vi "PW_LDA analysis top level_PN.vi"() -> ()   [LabVIEW 2010]
uses:
  PW_LDA control cluster.ctl
  PW_LDA wrapper control cluster.ctl
  <vilib>/Utility/file.llb/Read From Spreadsheet File (string).vi
panel:
  out "Correl files creation error":errorcluster
  out "Correl files writing / closing error":errorcluster
  out "stats file error":errorcluster
  out "Final error":errorcluster
  out "No. of rows":i32=67
  in  "Stats output directory":path=path "C:/LDAPW data/5ms_stats"
  out "Current row no.":i32=2
  in  "Wrapper controls":T1={"N blocks"=20, "PW lag time start (s)"=-0.2, "PW lag time finish (s)"=0.2, "PW lag time dt (s)"=0.2, "Desired lag time for stats (s)"=0.0, "stats order"=4, "PDF(T) or hist(F)"=TRUE, "Nbins U"=32, "Nbins V"=32, "Mean shift"=FALSE, "2nd comp."="v"}
  out "Batch file":string[][](array[string])=[["Block data path", "Output directory for lagged correls.", "X (mm)", "Y (mm)", "N blocks"], ["NEXT", "C:\\LDAPW data\\x=0_5ms", "", "", ""], ["C:\\LDAPW data\\x=0, y=0.5 5ms", "C:\\LDAPW data\\x=0_5ms", "0", "0.5", "20"], ["C:\\LDAPW data\\x=0, y=0.79 5ms", "C:\\LDAPW data\\x=0_5ms", "0", "0.79", "20"], ["C:\\LDAPW data\\x=0, y=1.23 5ms", "C:\\LDAPW data\\x=0_5ms", "0", "1.23", "20"], ["C:\\LDAPW data\\x=0, y=1.94 5ms", "C:\\LDAPW data\\x=0_5ms", "0", "1.94", "20"], ["C:\\LDAPW data\\x=0, y=3.04 5ms", "C:\\LDAPW data\\x=0_5ms", "0", "3.04", "20"], ["C:\\LDAPW data\\x=0, y=4.78 5ms", "C:\\LDAPW data\\x=0_5ms", "0", "4.78", "20"], ["C:\\LDAPW data\\x=0, y=7.5 5ms", "C:\\LDAPW data\\x=0_5ms", "0", "7.5", "20"], ["NEXT", "C:\\LDAPW data\\x=20_5ms", "", "", ""], ["C:\\LDAPW data\\x=20, y=0.5 5ms", "C:\\LDAPW data\\x=20_5ms", "20", "0.5", "20"], ["C:\\LDAPW data\\x=20, y=0.79 5ms", "C:\\LDAPW data\\x=20_5ms", "20", "0.79", "20"], ["C:\\LDAPW data\\x=20, y=1.23 5ms", "C:\\LDAPW data\\x=20_5ms", "20", "1.23", "20"], ["C:\\LDAPW data\\x=20, y=1.94 5ms", "C:\\LDAPW data\\x=20_5ms", "20", "1.94", "20"], ["C:\\LDAPW data\\x=20, y=3.04 5ms", "C:\\LDAPW data\\x=20_5ms", "20", "3.04", "20"], ["C:\\LDAPW data\\x=20, y=4.78 5ms", "C:\\LDAPW data\\x=20_5ms", "20", "4.78", "20"], ["C:\\LDAPW data\\x=20, y=7.5 5ms", "C:\\LDAPW data\\x=20_5ms", "20", "7.5", "20"], ["NEXT", "C:\\LDAPW data\\x=40_5ms", "", "", ""], ["C:\\LDAPW data\\x=40, y=0.55 5ms", "C:\\LDAPW data\\x=40_5ms", "40", "0.55", "20"], ["C:\\LDAPW data\\x=40, y=0.79 5ms", "C:\\LDAPW data\\x=40_5ms", "40", "0.79", "20"], ["C:\\LDAPW data\\x=40, y=1.23 5ms", "C:\\LDAPW data\\x=40_5ms", "40", "1.23", "20"], ["C:\\LDAPW data\\x=40, y=1.94 5ms", "C:\\LDAPW data\\x=40_5ms", "40", "1.94", "20"], ["C:\\LDAPW data\\x=40, y=3.04 5ms", "C:\\LDAPW data\\x=40_5ms", "40", "3.04", "20"], ["C:\\LDAPW data\\x=40, y=4.78 5ms", "C:\\LDAPW data\\x=40_5ms", "40", "4.78", "20"], ["C:\\LDAPW data\\x=40, y=7.5 5ms", "C:\\LDAPW data\\x=40_5ms", "40", "7.5", "20"], ["NEXT", "C:\\LDAPW data\\x=60_5ms", "", "", ""], ["C:\\LDAPW data\\x=60, y=0.5 5ms", "C:\\LDAPW data\\x=60_5ms", "60", "0.5", "20"], ["C:\\LDAPW data\\x=60, y=0.79 5ms", "C:\\LDAPW data\\x=60_5ms", "60", "0.79", "20"], ["C:\\LDAPW data\\x=60, y=1.23 5ms", "C:\\LDAPW data\\x=60_5ms", "60", "1.23", "20"], ["C:\\LDAPW data\\x=60, y=1.94 5ms", "C:\\LDAPW data\\x=60_5ms", "60", "1.94", "20"], ["C:\\LDAPW data\\x=60, y=3.04 5ms", "C:\\LDAPW data\\x=60_5ms", "60", "3.04", "20"], ["C:\\LDAPW data\\x=60, y=4.78 5ms", "C:\\LDAPW data\\x=60_5ms", "60", "4.78", "20"], ["C:\\LDAPW data\\x=60, y=7.5 5ms", "C:\\LDAPW data\\x=60_5ms", "60", "7.5", "20"], ["NEXT", "C:\\LDAPW data\\x=80_5ms", "", "", ""], ["C:\\LDAPW data\\x=80, y=0.5 5ms", "C:\\LDAPW data\\x=80_5ms", "80", "0.5", "20"], ["C:\\LDAPW data\\x=80, y=0.79 5ms", "C:\\LDAPW data\\x=80_5ms", "80", "0.79", "20"], ["C:\\LDAPW data\\x=80, y=1.23 5ms", "C:\\LDAPW data\\x=80_5ms", "80", "1.23", "20"], ["C:\\LDAPW data\\x=80, y=1.94 5ms", "C:\\LDAPW data\\x=80_5ms", "80", "1.94", "20"], ["C:\\LDAPW data\\x=80, y=3.04 5ms", "C:\\LDAPW data\\x=80_5ms", "80", "3.04", "20"], ["C:\\LDAPW data\\x=80, y=4.78 5ms", "C:\\LDAPW data\\x=80_5ms", "80", "4.78", "20"], ["C:\\LDAPW data\\x=80, y=7.5 5ms", "C:\\LDAPW data\\x=80_5ms", "80", "7.5", "20"], ["NEXT", "C:\\LDAPW data\\x=100_5ms", "", "", ""], ["C:\\LDAPW data\\x=100, y=0.5 5ms", "C:\\LDAPW data\\x=100_5ms", "100", "0.5", "20"], ["C:\\LDAPW data\\x=100, y=0.79 5ms", "C:\\LDAPW data\\x=100_5ms", "100", "0.79", "20"], ["C:\\LDAPW data\\x=100, y=1.23 5ms", "C:\\LDAPW data\\x=100_5ms", "100", "1.23", "20"], ["C:\\LDAPW data\\x=100, y=1.94 5ms", "C:\\LDAPW data\\x=100_5ms", "100", "1.94", "20"], ["C:\\LDAPW data\\x=100, y=3.04 5ms", "C:\\LDAPW data\\x=100_5ms", "100", "3.04", "20"], ["C:\\LDAPW data\\x=100, y=4.78 5ms", "C:\\LDAPW data\\x=100_5ms", "100", "4.78", "20"], ["C:\\LDAPW data\\x=100, y=7.5 5ms", "C:\\LDAPW data\\x=100_5ms", "100", "7.5", "20"], ["NEXT", "C:\\LDAPW data\\x=120_5ms", "", "", ""], ["C:\\LDAPW data\\x=120, y=0.5 5ms", "C:\\LDAPW data\\x=120_5ms", "120", "0.5", "20"], ["C:\\LDAPW data\\x=120, y=0.79 5ms", "C:\\LDAPW data\\x=120_5ms", "120", "0.79", "20"], ["C:\\LDAPW data\\x=120, y=1.23 5ms", "C:\\LDAPW data\\x=120_5ms", "120", "1.23", "20"], ["C:\\LDAPW data\\x=120, y=1.94 5ms", "C:\\LDAPW data\\x=120_5ms", "120", "1.94", "20"], ["C:\\LDAPW data\\x=120, y=3.04 5ms", "C:\\LDAPW data\\x=120_5ms", "120", "3.04", "20"], ["C:\\LDAPW data\\x=120, y=4.78 5ms", "C:\\LDAPW data\\x=120_5ms", "120", "4.78", "20"], ["C:\\LDAPW data\\x=120, y=7.5 5ms", "C:\\LDAPW data\\x=120_5ms", "120", "7.5", "20"], ["NEXT", "C:\\LDAPW data\\x=140_5ms", "", "", ""], ["C:\\LDAPW data\\x=140, y=0.5 5ms", "C:\\LDAPW data\\x=140_5ms", "140", "0.5", "20"], ["C:\\LDAPW data\\x=140, y=0.79 5ms", "C:\\LDAPW data\\x=140_5ms", "140", "0.79", "20"], ["C:\\LDAPW data\\x=140, y=1.23 5ms", "C:\\LDAPW data\\x=140_5ms", "140", "1.23", "20"], ["C:\\LDAPW data\\x=140, y=1.94 5ms", "C:\\LDAPW data\\x=140_5ms", "140", "1.94", "20"], ["C:\\LDAPW data\\x=140, y=3.04 5ms", "C:\\LDAPW data\\x=140_5ms", "140", "3.04", "20"], ["C:\\LDAPW data\\x=140, y=4.78 5ms", "C:\\LDAPW data\\x=140_5ms", "140", "4.78", "20"], ["C:\\LDAPW data\\x=140, y=7.5 5ms", "C:\\LDAPW data\\x=140_5ms", "140", "7.5", "20"], ["NEXT", "C:\\LDAPW data\\x=161.5_5ms", "", "", ""], ["C:\\LDAPW data\\x=161.5, y=0.53 5ms", "C:\\LDAPW data\\x=161.5_5ms", "161.5", "0.53", "20"], ["C:\\LDAPW data\\x=161.5, y=0.79 5ms", "C:\\LDAPW data\\x=161.5_5ms", "161.5", "0.79", "2"]]
  in  "Batch-file name":path=path "C:/LDAPW data/Full DataList.txt"
  in  "PW_LDA control cluster":T2={"Block data directory"=path "C:/LDAPW data/x=0, y=0.5 5ms", "An samp. rate (Hz)"=5000.0, "PW sampling rate (Hz)"=10.0, "PW samples per block"=300, "High threshold (V)"=2.5, "An. data prefix"="Analogue_", "LDA data prefix"="LDA_", "PW data prefix"="PW_", "LDA arr. t. prefix"="LDA_arr_t_", "filename suffix"=".txt", "interp. method"=1, "PW hardware delay (s)"=0.00085, "PW timing TOF fraction (0..1)"=0.5, "- LDA V"=TRUE, "PW TOF prefix"="PW_TOF_", "- LDA U"=FALSE, "- PW"=FALSE, "format"="%.16f"} {"interp. method" items=["nearest", "linear", "spline", "cubic Hermite", "Lagrange"]}
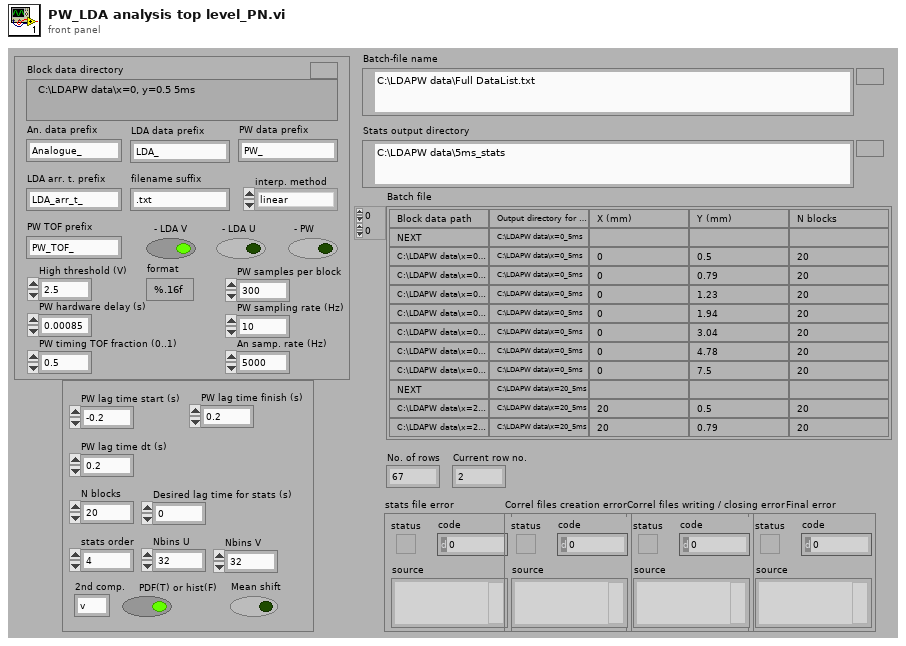
[diagram p1: front panel]
types:
  T1 = typedef "PW_LDA wrapper control cluster.ctl" = cluster{"N blocks":i32, "PW lag time start (s)":dbl, "PW lag time finish (s)":dbl, "PW lag time dt (s)":dbl, "Desired lag time for stats (s)":dbl, "stats order":i32, "PDF(T) or hist(F)":bool, "Nbins U":i32, "Nbins V":i32, "Mean shift":bool, "2nd comp.":string}
  T2 = typedef "PW_LDA control cluster.ctl" = cluster{"Block data directory":path, "An samp. rate (Hz)":dbl, "PW sampling rate (Hz)":dbl, "PW samples per block":i32, "High threshold (V)":dbl, "An. data prefix":string, "LDA data prefix":string, "PW data prefix":string, "LDA arr. t. prefix":string, "filename suffix":string, "interp. method":i32, "PW hardware delay (s)":dbl, "PW timing TOF fraction (0..1)":dbl, "- LDA V":bool, "PW TOF prefix":string, "- LDA U":bool, "- PW":bool, "format":string}
  T3 = enum16{"open", "replace", "create", "open or create", "replace or create", "replace or create with confirmation"}
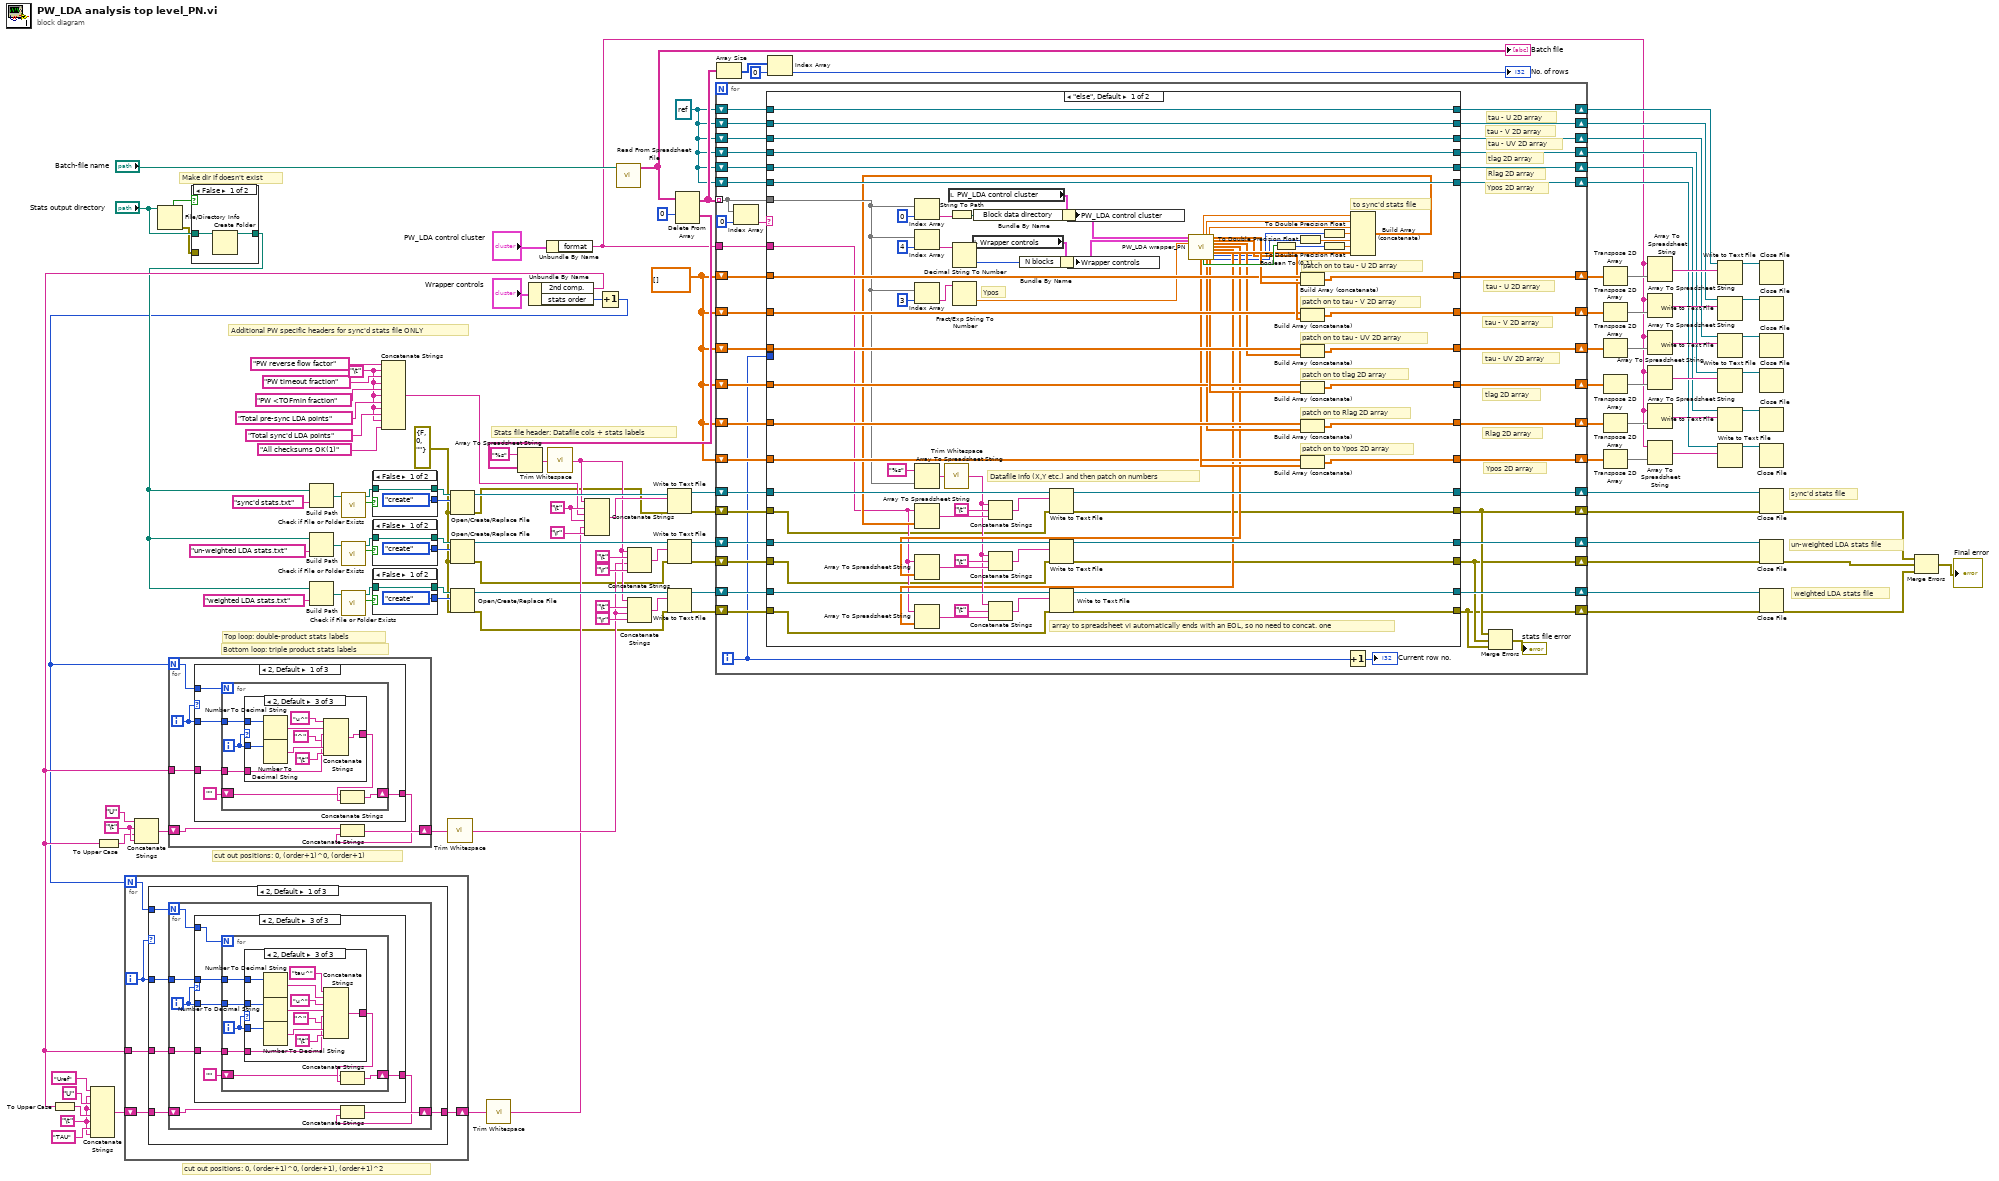
[diagram p0: block diagram]
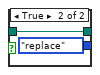
[diagram p3: hidden frame]
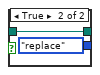
[diagram p4: hidden frame]
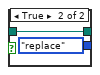
[diagram p5: hidden frame]
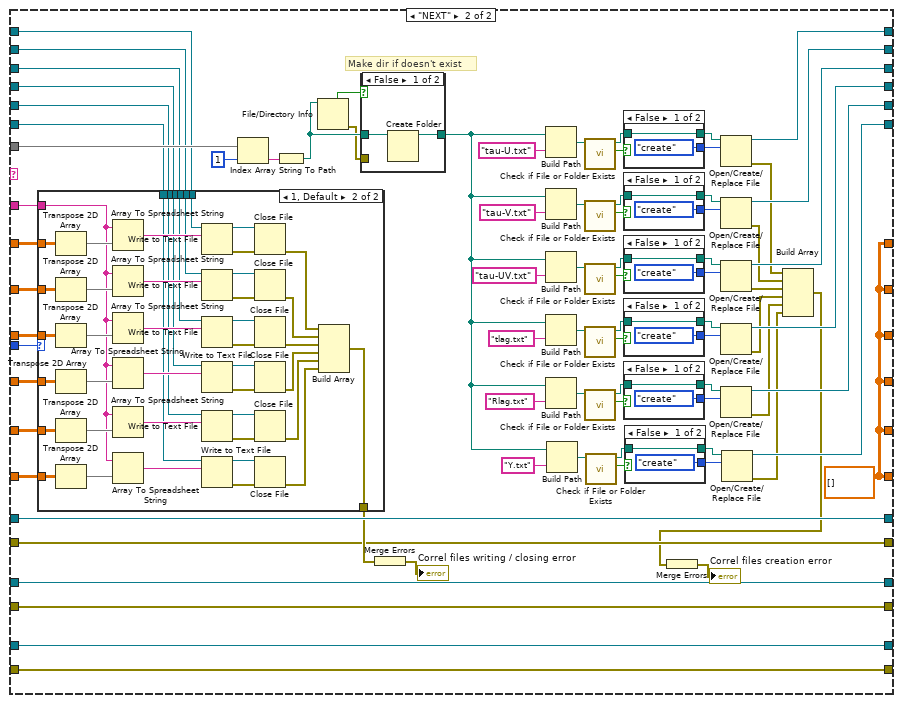
[diagram p6: hidden frame]
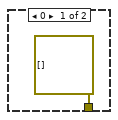
[diagram p8: hidden frame]
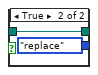
[diagram p9: hidden frame]
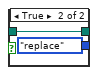
[diagram p10: hidden frame]
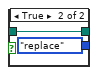
[diagram p11: hidden frame]
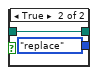
[diagram p12: hidden frame]
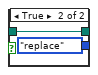
[diagram p13: hidden frame]
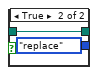
[diagram p14: hidden frame]
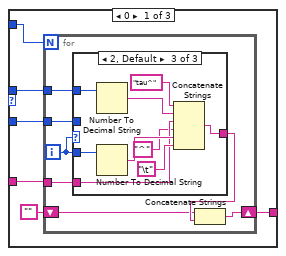
[diagram p15: hidden frame]
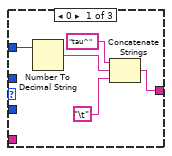
[diagram p16: hidden frame]
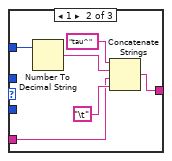
[diagram p17: hidden frame]
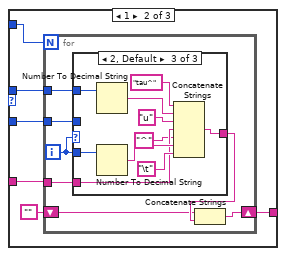
[diagram p18: hidden frame]
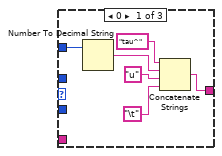
[diagram p19: hidden frame]
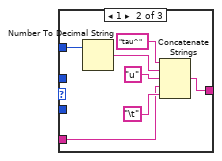
[diagram p20: hidden frame]
diagram:
  w14 = errorcluster {"status"=FALSE, "code"=0, "source"=""} ("error in")
  w64 = "\t"
  w70 = "\t"
  w112 = refnum<file> refnum ("refnum out")
  w111 = dbl[][] []
  w2 = "\t"
  w124 = "\t"
  # "Make dir if doesn't exist"
  # "Additional PW specific headers for sync'd stats file ONLY"
  # "Bottom loop: triple product stats labels"
  # "Top loop: double-product stats labels"
  # "Stats file header: Datafile cols + stats labels"
  # "weighted LDA stats file"
  # "un-weighted LDA stats file"
  # "sync'd stats file"
  # "cut out positions: 0, (order+1)^0, (order+1), (order+1)^2"
  # "cut out positions: 0, (order+1)^0, (order+1)"
  n1 = File/Directory Info(path="Stats output directory") -> (directory=w10:bool, error out=w7:errorcluster)  [unwired: 1 in, 5 out]
  n2 = case shown="False" w10 {
    tunnel: "Stats output directory" -> [w127 w128]
    tunnel: [w126 w128] -> w8
    tunnel: w7 -> [_ _]
    frame False {
      n3 = Create Folder(path (use dialog)=w127) -> (created path=w126:path)  [unwired: 1 in, 3 out]
    }
    frame True {
    }
  }
  n4 = Build Path(base path=w8, name or relative path="sync'd stats.txt" ("format string")) -> (appended path=w13:path)
  n5 = Build Path(base path=w8, name or relative path="un-weighted LDA stats.txt" ("format string")) -> (appended path=w12:path)
  n6 = Build Path(base path=w8, name or relative path="weighted LDA stats.txt" ("format string")) -> (appended path=w11:path)
  n7 = call <vilib>:"Check if File or Folder Exists.vi"("path"=w13) -> ("file or folder exists?"=w106:bool, "dup path"=w104:path)  [unwired: 1 in, 8 out]
  n8 = call <vilib>:"Check if File or Folder Exists.vi"("path"=w12) -> ("file or folder exists?"=w99:bool, "dup path"=w101:path)  [unwired: 1 in, 8 out]
  n9 = call <vilib>:"Check if File or Folder Exists.vi"("path"=w11) -> ("file or folder exists?"=w96:bool, "dup path"=w94:path)  [unwired: 1 in, 8 out]
  n10 = case shown="False" w106 {
    tunnel: [T3."create" ("operation (0:open)") T3."replace" ("operation (0:open)")] -> w105
    tunnel: [w129 w131] -> w103
    tunnel: w104 -> [w129 w131]
    frame False {
    }
    frame True {
    }
  }
  n11 = case shown="False" w99 {
    tunnel: [T3."create" ("operation (0:open)") T3."replace" ("operation (0:open)")] -> w100
    tunnel: [w133 w135] -> w102
    tunnel: w101 -> [w133 w135]
    frame False {
    }
    frame True {
    }
  }
  n12 = case shown="False" w96 {
    tunnel: [T3."create" ("operation (0:open)") T3."replace" ("operation (0:open)")] -> w95
    tunnel: [w137 w139] -> w93
    tunnel: w94 -> [w137 w139]
    frame False {
    }
    frame True {
    }
  }
  n13 = Concatenate Strings("PW reverse flow factor" ("format string"), w64, "PW timeout fraction" ("format string"), w64, "PW <TOFmin fraction" ("format string"), w64, "Total pre-sync LDA points" ("format string"), w64, "Total sync'd LDA points" ("format string"), w64, "All checksums OK(1)" ("format string")) -> (w62:string)
  n14 = Open/Create/Replace File(file path (use dialog)=w103, error in=w14, operation (0:open)=w105) -> (refnum out=w78:refnum<file>, error out=w59:errorcluster)  [unwired: 4 out]
  n15 = Open/Create/Replace File(file path (use dialog)=w102, error in=w14, operation (0:open)=w100) -> (refnum out=w77:refnum<file>, error out=w60:errorcluster)  [unwired: 4 out]
  n16 = Open/Create/Replace File(file path (use dialog)=w93, error in=w14, operation (0:open)=w95) -> (refnum out=w76:refnum<file>, error out=w61:errorcluster)  [unwired: 4 out]
  n17 = Unbundle By Name("Wrapper controls") -> ("2nd comp."=w108:string, "stats order"=w6:i32)
  n18 = To Upper Case(1:w108) -> (0:w4:string)
  n19 = Concatenate Strings("Uref" ("string"), w2, "U" ("string"), w2, w4, w2, "TAU" ("string"), w2) -> (w121:string)
  n20 = To Upper Case(1:w108) -> (0:w122:string)
  n21 = Concatenate Strings("U" ("string"), w124, w122, w124) -> (w123:string)
  n22 = Unbundle By Name("PW_LDA control cluster") -> ("format"=w22:string)
  n23 = Increment(x=w6) -> (x+1=w5:i32)
  n24 = for {
    N: w5 -> [w143]
    tunnel: w108 -> [w145]
    shift-right: [w144] -> w72
    shift-left: w121 -> [w142]
    i -> [w141]
    n25 = case shown="2, Default" w141 {
      tunnel: w145 -> [w150 w273 w363]
      tunnel: [w149 w272 w362] -> w144
      tunnel: w143 -> [w148 w271 w361]
      tunnel: w142 -> [w147 w270 w360]
      tunnel: w141 -> [w146 w269 w359]
      frame 2, Default {
        n26 = for {
          N: w148 -> [w157]
          shift-right: [w156] -> w149
          shift-left: w147 -> [w155]
          tunnel: w150 -> [w153]
          tunnel: w146 -> [w151]
          i -> [w152]
          n27 = case shown="2, Default" w152 {
            tunnel: w157 -> [w163 w196 w232]
            tunnel: [w161 w194 w230] -> w154
            tunnel: w153 -> [w160 w193 w229]
            tunnel: w152 -> [w159 w192 w228]
            tunnel: w151 -> [w158 w191 w227]
            frame 0 {
              n28 = for {
                N: w163 -> [_]
                shift-right: [w169] -> w161
                shift-left: "" -> [w168]
                tunnel: w159 -> [w167]
                tunnel: w160 -> [w166]
                tunnel: w158 -> [w164]
                i -> [w165]
                n29 = case shown="2, Default" w165 {
                  tunnel: [w175 w181 w190] -> w170
                  tunnel: w167 -> [_ _ _]
                  tunnel: w166 -> [_ w179 w187]
                  tunnel: w165 -> [_ _ w186]
                  tunnel: w164 -> [w173 w177 w184]
                  frame 0 {
                    n30 = Number To Decimal String(number=w173) -> (decimal integer string=w172:string)  [unwired: 1 out]
                    n31 = Concatenate Strings("tau^" ("t"), w172, "\t") -> (w175:string)
                  }
                  frame 1 {
                    n32 = Number To Decimal String(number=w177) -> (decimal integer string=w176:string)  [unwired: 1 out]
                    n33 = Concatenate Strings("tau^" ("t"), w176, w179, "\t") -> (w181:string)
                  }
                  frame 2, Default {
                    n34 = Number To Decimal String(number=w184) -> (decimal integer string=w183:string)  [unwired: 1 out]
                    n35 = Number To Decimal String(number=w186) -> (decimal integer string=w189:string)  [unwired: 1 out]
                    n36 = Concatenate Strings("tau^" ("t"), w183, w187, "^" ("string"), w189, "\t") -> (w190:string)
                  }
                }
                n37 = Concatenate Strings(w168, w170) -> (w169:string)
              }
            }
            frame 1 {
              n38 = for {
                N: w196 -> [_]
                shift-right: [w202] -> w194
                shift-left: "" -> [w201]
                tunnel: w192 -> [w200]
                tunnel: w193 -> [w199]
                tunnel: w191 -> [w197]
                i -> [w198]
                n39 = case shown="2, Default" w198 {
                  tunnel: [w208 w215 w225] -> w203
                  tunnel: w200 -> [_ _ _]
                  tunnel: w199 -> [_ w213 w222]
                  tunnel: w198 -> [_ _ w221]
                  tunnel: w197 -> [w206 w211 w219]
                  frame 0 {
                    n40 = Number To Decimal String(number=w206) -> (decimal integer string=w205:string)  [unwired: 1 out]
                    n41 = Concatenate Strings("tau^" ("t"), w205, "u" ("t"), "\t") -> (w208:string)
                  }
                  frame 1 {
                    n42 = Number To Decimal String(number=w211) -> (decimal integer string=w210:string)  [unwired: 1 out]
                    n43 = Concatenate Strings("tau^" ("t"), w210, "u" ("t"), w213, "\t") -> (w215:string)
                  }
                  frame 2, Default {
                    n44 = Number To Decimal String(number=w219) -> (decimal integer string=w218:string)  [unwired: 1 out]
                    n45 = Number To Decimal String(number=w221) -> (decimal integer string=w224:string)  [unwired: 1 out]
                    n46 = Concatenate Strings("tau^" ("t"), w218, "u" ("t"), w222, "^" ("string"), w224, "\t") -> (w225:string)
                  }
                }
                n47 = Concatenate Strings(w201, w203) -> (w202:string)
              }
            }
            frame 2, Default {
              n48 = for {
                N: w232 -> [_]
                shift-right: [w238] -> w230
                shift-left: "" -> [w237]
                tunnel: w228 -> [w236]
                tunnel: w229 -> [w235]
                tunnel: w227 -> [w233]
                i -> [w234]
                n49 = case shown="2, Default" w234 {
                  tunnel: [w246 w255 w267] -> w239
                  tunnel: w236 -> [w244 w253 w264]
                  tunnel: w235 -> [_ w251 w262]
                  tunnel: w234 -> [_ _ w261]
                  tunnel: w233 -> [w242 w249 w259]
                  frame 0 {
                    n50 = Number To Decimal String(number=w242) -> (decimal integer string=w241:string)  [unwired: 1 out]
                    n51 = Number To Decimal String(number=w244) -> (decimal integer string=w245:string)  [unwired: 1 out]
                    n52 = Concatenate Strings("tau^" ("t"), w241, "u^" ("t"), w245, "\t") -> (w246:string)
                  }
                  frame 1 {
                    n53 = Number To Decimal String(number=w249) -> (decimal integer string=w248:string)  [unwired: 1 out]
                    n54 = Number To Decimal String(number=w253) -> (decimal integer string=w254:string)  [unwired: 1 out]
                    n55 = Concatenate Strings("tau^" ("t"), w248, "u^" ("t"), w254, w251, "\t") -> (w255:string)
                  }
                  frame 2, Default {
                    n56 = Number To Decimal String(number=w259) -> (decimal integer string=w258:string)  [unwired: 1 out]
                    n57 = Number To Decimal String(number=w264) -> (decimal integer string=w266:string)  [unwired: 1 out]
                    n58 = Number To Decimal String(number=w261) -> (decimal integer string=w265:string)  [unwired: 1 out]
                    n59 = Concatenate Strings("tau^" ("t"), w258, "u^" ("t"), w266, w262, "^" ("string"), w265, "\t") -> (w267:string)
                  }
                }
                n60 = Concatenate Strings(w237, w239) -> (w238:string)
              }
            }
          }
          n61 = Concatenate Strings(w155, w154) -> (w156:string)
        }
      }
      frame 0 {
        n62 = for {
          N: w271 -> [w280]
          shift-right: [w279] -> w272
          shift-left: w270 -> [w278]
          tunnel: w273 -> [w276]
          tunnel: w269 -> [w274]
          i -> [w275]
          n63 = case shown="2, Default" w275 {
            tunnel: w280 -> [w286 w306 w331]
            tunnel: [w284 w304 w329] -> w277
            tunnel: w276 -> [w283 w303 w328]
            tunnel: w275 -> [w282 w302 w327]
            tunnel: w274 -> [w281 w301 w326]
            frame 0 {
              n64 = for {
                N: w286 -> [_]
                shift-right: [w292] -> w284
                shift-left: "" -> [w291]
                tunnel: w282 -> [w290]
                tunnel: w283 -> [w289]
                tunnel: w281 -> [w287]
                i -> [w288]
                n65 = case shown="2, Default" w288 {
                  tunnel: ["" w300] -> w293
                  tunnel: w290 -> [_ _]
                  tunnel: w289 -> [_ w297]
                  tunnel: w288 -> [_ w296]
                  tunnel: w287 -> [_ _]
                  frame 0, 1 {
                  }
                  frame 2, Default {
                    n66 = Number To Decimal String(number=w296) -> (decimal integer string=w299:string)  [unwired: 1 out]
                    n67 = Concatenate Strings(w297, "^" ("string"), w299, "\t") -> (w300:string)
                  }
                }
                n68 = Concatenate Strings(w291, w293) -> (w292:string)
              }
            }
            frame 1 {
              n69 = for {
                N: w306 -> [_]
                shift-right: [w312] -> w304
                shift-left: "" -> [w311]
                tunnel: w302 -> [w310]
                tunnel: w303 -> [w309]
                tunnel: w301 -> [w307]
                i -> [w308]
                n70 = case shown="2, Default" w308 {
                  tunnel: ["" w317 w324] -> w313
                  tunnel: w310 -> [_ _ _]
                  tunnel: w309 -> [_ w315 w321]
                  tunnel: w308 -> [_ _ w320]
                  tunnel: w307 -> [_ _ _]
                  frame 0 {
                  }
                  frame 1 {
                    n71 = Concatenate Strings("u" ("t"), w315, "\t") -> (w317:string)
                  }
                  frame 2, Default {
                    n72 = Number To Decimal String(number=w320) -> (decimal integer string=w323:string)  [unwired: 1 out]
                    n73 = Concatenate Strings("u" ("t"), w321, "^" ("string"), w323, "\t") -> (w324:string)
                  }
                }
                n74 = Concatenate Strings(w311, w313) -> (w312:string)
              }
            }
            frame 2, Default {
              n75 = for {
                N: w331 -> [_]
                shift-right: [w337] -> w329
                shift-left: "" -> [w336]
                tunnel: w327 -> [w335]
                tunnel: w328 -> [w334]
                tunnel: w326 -> [w332]
                i -> [w333]
                n76 = case shown="2, Default" w333 {
                  tunnel: [w342 w348 w357] -> w338
                  tunnel: w335 -> [w340 w346 w354]
                  tunnel: w334 -> [_ w344 w352]
                  tunnel: w333 -> [_ _ w351]
                  tunnel: w332 -> [_ _ _]
                  frame 0 {
                    n77 = Number To Decimal String(number=w340) -> (decimal integer string=w341:string)  [unwired: 1 out]
                    n78 = Concatenate Strings("u^" ("t"), w341, "\t") -> (w342:string)
                  }
                  frame 1 {
                    n79 = Number To Decimal String(number=w346) -> (decimal integer string=w347:string)  [unwired: 1 out]
                    n80 = Concatenate Strings("u^" ("t"), w347, w344, "\t") -> (w348:string)
                  }
                  frame 2, Default {
                    n81 = Number To Decimal String(number=w354) -> (decimal integer string=w356:string)  [unwired: 1 out]
                    n82 = Number To Decimal String(number=w351) -> (decimal integer string=w355:string)  [unwired: 1 out]
                    n83 = Concatenate Strings("u^" ("t"), w356, w352, "^" ("string"), w355, "\t") -> (w357:string)
                  }
                }
                n84 = Concatenate Strings(w336, w338) -> (w337:string)
              }
            }
          }
          n85 = Concatenate Strings(w278, w277) -> (w279:string)
        }
      }
      frame 1 {
        n86 = for {
          N: w361 -> [w370]
          shift-right: [w369] -> w362
          shift-left: w360 -> [w368]
          tunnel: w363 -> [w366]
          tunnel: w359 -> [w364]
          i -> [w365]
          n87 = case shown="2, Default" w365 {
            tunnel: w370 -> [w376 w401 w431]
            tunnel: [w375 w399 w429] -> w367
            tunnel: w366 -> [w374 w398 w428]
            tunnel: w365 -> [w373 w397 w427]
            tunnel: w364 -> [w372 w396 w426]
            frame 0 {
              n88 = for {
                N: w376 -> [_]
                shift-right: [w382] -> w375
                shift-left: "" -> [w381]
                tunnel: w373 -> [w380]
                tunnel: w374 -> [w379]
                tunnel: w372 -> [w377]
                i -> [w378]
                n89 = case shown="2, Default" w378 {
                  tunnel: ["" w388 w395] -> w383
                  tunnel: w380 -> [_ _ _]
                  tunnel: w379 -> [_ w386 w392]
                  tunnel: w378 -> [_ _ w391]
                  tunnel: w377 -> [_ _ _]
                  frame 0 {
                  }
                  frame 1 {
                    n90 = Concatenate Strings("tau" ("t"), w386, "\t") -> (w388:string)
                  }
                  frame 2, Default {
                    n91 = Number To Decimal String(number=w391) -> (decimal integer string=w394:string)  [unwired: 1 out]
                    n92 = Concatenate Strings("tau" ("t"), w392, "^" ("string"), w394, "\t") -> (w395:string)
                  }
                }
                n93 = Concatenate Strings(w381, w383) -> (w382:string)
              }
            }
            frame 1 {
              n94 = for {
                N: w401 -> [_]
                shift-right: [w407] -> w399
                shift-left: "" -> [w406]
                tunnel: w397 -> [w405]
                tunnel: w398 -> [w404]
                tunnel: w396 -> [w402]
                i -> [w403]
                n95 = case shown="2, Default" w403 {
                  tunnel: [w411 w416 w424] -> w408
                  tunnel: w405 -> [_ _ _]
                  tunnel: w404 -> [_ w414 w421]
                  tunnel: w403 -> [_ _ w420]
                  tunnel: w402 -> [_ _ _]
                  frame 0 {
                    n96 = Concatenate Strings("tau" ("t"), "u" ("t"), "\t") -> (w411:string)
                  }
                  frame 1 {
                    n97 = Concatenate Strings("tau" ("t"), "u" ("t"), w414, "\t") -> (w416:string)
                  }
                  frame 2, Default {
                    n98 = Number To Decimal String(number=w420) -> (decimal integer string=w423:string)  [unwired: 1 out]
                    n99 = Concatenate Strings("tau" ("t"), "u" ("t"), w421, "^" ("string"), w423, "\t") -> (w424:string)
                  }
                }
                n100 = Concatenate Strings(w406, w408) -> (w407:string)
              }
            }
            frame 2, Default {
              n101 = for {
                N: w431 -> [_]
                shift-right: [w437] -> w429
                shift-left: "" -> [w436]
                tunnel: w427 -> [w435]
                tunnel: w428 -> [w434]
                tunnel: w426 -> [w432]
                i -> [w433]
                n102 = case shown="2, Default" w433 {
                  tunnel: [w443 w450 w460] -> w438
                  tunnel: w435 -> [w441 w448 w457]
                  tunnel: w434 -> [_ w446 w455]
                  tunnel: w433 -> [_ _ w454]
                  tunnel: w432 -> [_ _ _]
                  frame 0 {
                    n103 = Number To Decimal String(number=w441) -> (decimal integer string=w442:string)  [unwired: 1 out]
                    n104 = Concatenate Strings("tau" ("t"), "u^" ("t"), w442, "\t") -> (w443:string)
                  }
                  frame 1 {
                    n105 = Number To Decimal String(number=w448) -> (decimal integer string=w449:string)  [unwired: 1 out]
                    n106 = Concatenate Strings("tau" ("t"), "u^" ("t"), w449, w446, "\t") -> (w450:string)
                  }
                  frame 2, Default {
                    n107 = Number To Decimal String(number=w457) -> (decimal integer string=w459:string)  [unwired: 1 out]
                    n108 = Number To Decimal String(number=w454) -> (decimal integer string=w458:string)  [unwired: 1 out]
                    n109 = Concatenate Strings("tau" ("t"), "u^" ("t"), w459, w455, "^" ("string"), w458, "\t") -> (w460:string)
                  }
                }
                n110 = Concatenate Strings(w436, w438) -> (w437:string)
              }
            }
          }
          n111 = Concatenate Strings(w368, w367) -> (w369:string)
        }
      }
    }
  }
  n112 = for {
    N: w5 -> [w467]
    shift-right: [w466] -> w74
    shift-left: w123 -> [w465]
    tunnel: w108 -> [w463]
    i -> [w462]
    n113 = case shown="2, Default" w462 {
      tunnel: w467 -> [w472 w503 w521]
      tunnel: [w470 w501 w519] -> w464
      tunnel: w463 -> [w469 w500 w518]
      tunnel: w462 -> [w468 w499 w517]
      frame 2, Default {
        n114 = for {
          N: w472 -> [_]
          shift-right: [w477] -> w470
          shift-left: "" -> [w476]
          tunnel: w468 -> [w475]
          tunnel: w469 -> [w474]
          i -> [w473]
          n115 = case shown="2, Default" w473 {
            tunnel: [w482 w488 w497] -> w478
            tunnel: w475 -> [w480 w486 w494]
            tunnel: w474 -> [_ w484 w492]
            tunnel: w473 -> [_ _ w491]
            frame 0 {
              n116 = Number To Decimal String(number=w480) -> (decimal integer string=w481:string)  [unwired: 1 out]
              n117 = Concatenate Strings("u^" ("t"), w481, "\t") -> (w482:string)
            }
            frame 1 {
              n118 = Number To Decimal String(number=w486) -> (decimal integer string=w487:string)  [unwired: 1 out]
              n119 = Concatenate Strings("u^" ("t"), w487, w484, "\t") -> (w488:string)
            }
            frame 2, Default {
              n120 = Number To Decimal String(number=w494) -> (decimal integer string=w496:string)  [unwired: 1 out]
              n121 = Number To Decimal String(number=w491) -> (decimal integer string=w495:string)  [unwired: 1 out]
              n122 = Concatenate Strings("u^" ("t"), w496, w492, "^" ("string"), w495, "\t") -> (w497:string)
            }
          }
          n123 = Concatenate Strings(w476, w478) -> (w477:string)
        }
      }
      frame 0 {
        n124 = for {
          N: w503 -> [_]
          shift-right: [w508] -> w501
          shift-left: "" -> [w507]
          tunnel: w499 -> [w506]
          tunnel: w500 -> [w505]
          i -> [w504]
          n125 = case shown="2, Default" w504 {
            tunnel: ["" w516] -> w509
            tunnel: w506 -> [_ _]
            tunnel: w505 -> [_ w513]
            tunnel: w504 -> [_ w512]
            frame 0, 1 {
            }
            frame 2, Default {
              n126 = Number To Decimal String(number=w512) -> (decimal integer string=w515:string)  [unwired: 1 out]
              n127 = Concatenate Strings(w513, "^" ("string"), w515, "\t") -> (w516:string)
            }
          }
          n128 = Concatenate Strings(w507, w509) -> (w508:string)
        }
      }
      frame 1 {
        n129 = for {
          N: w521 -> [_]
          shift-right: [w526] -> w519
          shift-left: "" -> [w525]
          tunnel: w517 -> [w524]
          tunnel: w518 -> [w523]
          i -> [w522]
          n130 = case shown="2, Default" w522 {
            tunnel: ["" w531 w538] -> w527
            tunnel: w524 -> [_ _ _]
            tunnel: w523 -> [_ w529 w535]
            tunnel: w522 -> [_ _ w534]
            frame 0 {
            }
            frame 1 {
              n131 = Concatenate Strings("u" ("t"), w529, "\t") -> (w531:string)
            }
            frame 2, Default {
              n132 = Number To Decimal String(number=w534) -> (decimal integer string=w537:string)  [unwired: 1 out]
              n133 = Concatenate Strings("u" ("t"), w535, "^" ("string"), w537, "\t") -> (w538:string)
            }
          }
          n134 = Concatenate Strings(w525, w527) -> (w526:string)
        }
      }
    }
    n135 = Concatenate Strings(w465, w464) -> (w466:string)
  }
  n136 = call <vilib>:"Trim Whitespace.vi"("string"=w74) -> ("trimmed string"=w73:string)  [unwired: 1 in]
  n137 = call <vilib>:"Trim Whitespace.vi"("string"=w72) -> ("trimmed string"=w71:string)  [unwired: 1 in]
  n138 = call-poly <vilib>:"Read From Spreadsheet File.vi"("file path (dialog if empty)"="Batch-file name") -> ("all rows"=w118:string[][])  [unwired: 3 in, 7 out]
  "Batch file" <- w118
  n139 = Delete From Array(array=w118, index (row)=0) -> (deleted portion=w115:string[], array with subset deleted=w116:string[][])  [unwired: 2 in]
  n140 = Array To Spreadsheet String(array=w115, 3:"%s" ("format string")) -> (spreadsheet string=w113:string)  [unwired: 1 out]
  n141 = call <vilib>:"Trim Whitespace.vi"("string"=w113) -> ("trimmed string"=w75:string)  [unwired: 1 in]
  n142 = Concatenate Strings(w75, w70, w62, w70, w71, "\r") -> (w86:string)
  n143 = Concatenate Strings(w75, "\t", w73, "\r") -> (w80:string)
  n144 = Concatenate Strings(w75, "\t", w73, "\r") -> (w79:string)
  n145 = Write to Text File(file (use dialog)=w78, text=w86, error in=w59) -> (refnum out=w89:refnum<file>, error out=w56:errorcluster)  [unwired: 2 out]
  n146 = Write to Text File(file (use dialog)=w77, text=w80, error in=w60) -> (refnum out=w88:refnum<file>, error out=w57:errorcluster)  [unwired: 2 out]
  n147 = Write to Text File(file (use dialog)=w76, text=w79, error in=w61) -> (refnum out=w87:refnum<file>, error out=w58:errorcluster)  [unwired: 2 out]
  n148 = for {
    tunnel: w116 -> [w579] mode=indexing
    shift-right: [w578] -> w28
    shift-left: w112 -> [w577]
    shift-right: [w576] -> w33
    shift-left: w111 -> [w575]
    shift-right: [w574] -> w32
    shift-left: w111 -> [w573]
    shift-right: [w572] -> w31
    shift-left: w111 -> [w571]
    shift-right: [w570] -> w30
    shift-left: w111 -> [w569]
    shift-right: [w568] -> w21
    shift-left: w111 -> [w567]
    shift-right: [w566] -> w27
    shift-left: w112 -> [w565]
    shift-right: [w564] -> w26
    shift-left: w112 -> [w563]
    shift-right: [w562] -> w25
    shift-left: w112 -> [w561]
    shift-right: [w560] -> w24
    shift-left: w112 -> [w559]
    shift-right: [w558] -> w29
    shift-left: w111 -> [w557]
    shift-right: [w556] -> w23
    shift-left: w112 -> [w555]
    tunnel: w22 -> [w554]
    shift-right: [w550] -> w20
    shift-left: w89 -> [w553]
    shift-right: [w549] -> w18
    shift-left: w88 -> [w552]
    shift-right: [w548] -> w16
    shift-left: w87 -> [w551]
    shift-right: [w544] -> w19
    shift-left: w56 -> [w545]
    shift-right: [w543] -> w17
    shift-left: w57 -> [w546]
    shift-right: [w542] -> w15
    shift-left: w58 -> [w547]
    i -> [w540]
    # "Ypos 2D array"
    # "Rlag 2D array"
    # "tlag 2D array"
    # "tau - UV 2D array"
    # "tau - V 2D array"
    # "tau - U 2D array"
    # "Ypos 2D array"
    # "Rlag 2D array"
    # "tlag 2D array"
    # "tau - UV 2D array"
    # "tau - V 2D array"
    # "tau - U 2D array"
    n149 = Index Array(array=w579, index=0) -> (element=w581:string)
    n150 = case shown="\"else\", Default" w581 {
      tunnel: w579 -> [w618 w738]
      tunnel: [w625 w730] -> w578
      tunnel: w577 -> [w625 w688]
      tunnel: [w641 w681] -> w576
      tunnel: w575 -> [w640 w701]
      tunnel: [w638 w681] -> w574
      tunnel: w573 -> [w637 w697]
      tunnel: [w635 w681] -> w572
      tunnel: w571 -> [w636 w698]
      tunnel: [w633 w681] -> w570
      tunnel: w569 -> [w632 w699]
      tunnel: [w631 w681] -> w568
      tunnel: w567 -> [w630 w700]
      tunnel: [w624 w723] -> w566
      tunnel: w565 -> [w624 w687]
      tunnel: [w623 w716] -> w564
      tunnel: w563 -> [w623 w686]
      tunnel: [w622 w709] -> w562
      tunnel: w561 -> [w622 w685]
      tunnel: [w621 w702] -> w560
      tunnel: w559 -> [w621 w684]
      tunnel: [w627 w681] -> w558
      tunnel: w557 -> [w626 w696]
      tunnel: [w620 w689] -> w556
      tunnel: w555 -> [w620 w683]
      tunnel: w554 -> [w595 w682]
      tunnel: w553 -> [w613 w680]
      tunnel: w552 -> [w606 w679]
      tunnel: w551 -> [w599 w678]
      tunnel: [w612 w680] -> w550
      tunnel: [w605 w679] -> w549
      tunnel: [w598 w678] -> w548
      tunnel: w547 -> [w586 w668]
      tunnel: w546 -> [w587 w669]
      tunnel: w545 -> [w588 w670]
      tunnel: [w585 w668] -> w542
      tunnel: [w584 w669] -> w543
      tunnel: [w583 w670] -> w544
      tunnel: w540 -> [_ w664]
      frame "else", Default {
        # "array to spreadsheet vi automatically ends with an EOL, so no need to concat. one"
        # "Datafile info (X,Y etc.) and then patch on numbers"
        # "Ypos"
        # "patch on to Ypos 2D array"
        # "patch on to Rlag 2D array"
        # "patch on to tlag 2D array"
        # "patch on to tau - UV 2D array"
        # "patch on to tau - V 2D array"
        # "patch on to tau - U 2D array"
        # "to sync'd stats file"
        n151 = Index Array(array=w618, index=0) -> (element=w648:string)
        n152 = Index Array(array=w618, index=4) -> (element=w651:string)
        n153 = Index Array(array=w618, index=3) -> (element=w617:string)
        n154 = Array To Spreadsheet String(array=w618, 3:"%s" ("format string")) -> (spreadsheet string=w657:string)  [unwired: 1 out]
        n155 = call <vilib>:"Trim Whitespace.vi"("string"=w657) -> ("trimmed string"=w597:string)  [unwired: 1 in]
        n156 = local read "PW_LDA control cluster"() -> (w654:T2)
        n157 = String To Path(string=w648) -> (path=w650:path)
        n158 = Decimal String To Number(string=w651) -> (number=w649:i32)  [unwired: 3 out]
        n159 = Fract/Exp String To Number(string=w617) -> (number=w616:dbl)  [unwired: 4 out]
        n160 = local read "Wrapper controls"() -> (w652:T1)
        n161 = Bundle By Name(cluster=w654, "Block data directory"=w650) -> (w659:T2)
        n162 = Bundle By Name(cluster=w652, "N blocks"=w649) -> (w658:T1)
        n163 = local write "PW_LDA control cluster"(w659) -> ()
        n164 = local write "Wrapper controls"(w658) -> ()
        n165 = call "PW_LDA wrapper_PN.vi"("PW_LDA control cluster"=w659, "Wrapper controls"=w658, "Y pos"=w616) -> ("Y pos array"=w628:dbl[], "PW reverse flow factor"=w647:dbl, "All checksums okay"=w644:bool, "PW timeout fraction"=w646:dbl, "Rlag (m)"=w629:dbl[], "PW TOFmin cutoff fraction"=w645:dbl, "tlag (s)"=w634:dbl[], "Corr coeff. tau, U with PW lag time"=w642:dbl[], "Corr coeff. tau, V with PW lag time"=w639:dbl[], "Corr coeff. tau, UV with PW lag time"=w604:dbl[], "Un-weighted stats"=w603:dbl[], "Weighted stats"=w596:dbl[], "Sync'd stats"=w643:dbl[], "Total pre-sync LDA points"=w592:i32, "Total sync'd points"=w594:i32)  [unwired: 10 out]
        n166 = Array To Spreadsheet String(array=w603, 3:w595) -> (spreadsheet string=w608:string)  [unwired: 1 out]
        n167 = Array To Spreadsheet String(array=w596, 3:w595) -> (spreadsheet string=w600:string)  [unwired: 1 out]
        n168 = Concatenate Strings(w597, "\t", w608) -> (w607:string)
        n169 = Concatenate Strings(w597, "\t", w600) -> (w602:string)
        n170 = Write to Text File(file (use dialog)=w606, text=w607, error in=w587) -> (refnum out=w605:refnum<file>, error out=w584:errorcluster)  [unwired: 2 out]
        n171 = Write to Text File(file (use dialog)=w599, text=w602, error in=w586) -> (refnum out=w598:refnum<file>, error out=w585:errorcluster)  [unwired: 2 out]
        n172 = Boolean To (0,1)(Boolean=w644) -> (0, 1=w590:i16)
        n173 = To Double Precision Float(number=w594) -> (double precision float=w593:dbl)
        n174 = Build Array (concatenate)(w640, w642) -> (w641:dbl[][])
        n175 = Build Array (concatenate)(w637, w639) -> (w638:dbl[][])
        n176 = Build Array (concatenate)(w636, w604) -> (w635:dbl[][])
        n177 = Build Array (concatenate)(w632, w634) -> (w633:dbl[][])
        n178 = Build Array (concatenate)(w630, w629) -> (w631:dbl[][])
        n179 = Build Array (concatenate)(w626, w628) -> (w627:dbl[][])
        n180 = To Double Precision Float(number=w592) -> (double precision float=w591:dbl)
        n181 = To Double Precision Float(number=w590) -> (double precision float=w589:dbl)
        n182 = Build Array (concatenate)(w647, w646, w645, w591, w593, w589, w643) -> (w611:dbl[])
        n183 = Array To Spreadsheet String(array=w611, 3:w595) -> (spreadsheet string=w614:string)  [unwired: 1 out]
        n184 = Concatenate Strings(w597, "\t", w614) -> (w609:string)
        n185 = Write to Text File(file (use dialog)=w613, text=w609, error in=w588) -> (refnum out=w612:refnum<file>, error out=w583:errorcluster)  [unwired: 2 out]
      }
      frame "NEXT" {
        w681 = dbl[][] []
        # "Make dir if doesn't exist"
        n186 = case shown="1, Default" w664 {
          tunnel: w701 -> [_ w787]
          tunnel: w700 -> [_ w786]
          tunnel: w699 -> [_ w785]
          tunnel: w698 -> [_ w784]
          tunnel: w697 -> [_ w783]
          tunnel: w696 -> [_ w782]
          tunnel: w688 -> [_ w781]
          tunnel: w687 -> [_ w774]
          tunnel: w686 -> [_ w771]
          tunnel: w685 -> [_ w766]
          tunnel: w684 -> [_ w762]
          tunnel: w683 -> [_ w758]
          tunnel: w682 -> [_ w757]
          tunnel: [errorcluster[] [] w744] -> w671
          frame 0 {
          }
          frame 1, Default {
            n187 = Transpose 2D Array(2D array=w787) -> (transposed array=w780:dbl[][])
            n188 = Transpose 2D Array(2D array=w783) -> (transposed array=w775:dbl[][])
            n189 = Transpose 2D Array(2D array=w784) -> (transposed array=w772:dbl[][])
            n190 = Transpose 2D Array(2D array=w785) -> (transposed array=w767:dbl[][])
            n191 = Transpose 2D Array(2D array=w786) -> (transposed array=w763:dbl[][])
            n192 = Transpose 2D Array(2D array=w782) -> (transposed array=w759:dbl[][])
            n193 = Array To Spreadsheet String(array=w780, 3:w757) -> (spreadsheet string=w779:string)  [unwired: 1 out]
            n194 = Array To Spreadsheet String(array=w775, 3:w757) -> (spreadsheet string=w778:string)  [unwired: 1 out]
            n195 = Array To Spreadsheet String(array=w772, 3:w757) -> (spreadsheet string=w773:string)  [unwired: 1 out]
            n196 = Array To Spreadsheet String(array=w767, 3:w757) -> (spreadsheet string=w768:string)  [unwired: 1 out]
            n197 = Array To Spreadsheet String(array=w763, 3:w757) -> (spreadsheet string=w765:string)  [unwired: 1 out]
            n198 = Array To Spreadsheet String(array=w759, 3:w757) -> (spreadsheet string=w760:string)  [unwired: 1 out]
            n199 = Write to Text File(file (use dialog)=w781, text=w779) -> (refnum out=w777:refnum<file>, error out=w756:errorcluster)  [unwired: 1 in, 2 out]
            n200 = Write to Text File(file (use dialog)=w774, text=w778) -> (refnum out=w776:refnum<file>, error out=w755:errorcluster)  [unwired: 1 in, 2 out]
            n201 = Write to Text File(file (use dialog)=w771, text=w773) -> (refnum out=w770:refnum<file>, error out=w754:errorcluster)  [unwired: 1 in, 2 out]
            n202 = Write to Text File(file (use dialog)=w766, text=w768) -> (refnum out=w769:refnum<file>, error out=w753:errorcluster)  [unwired: 1 in, 2 out]
            n203 = Write to Text File(file (use dialog)=w762, text=w765) -> (refnum out=w764:refnum<file>, error out=w752:errorcluster)  [unwired: 1 in, 2 out]
            n204 = Write to Text File(file (use dialog)=w758, text=w760) -> (refnum out=w761:refnum<file>, error out=w751:errorcluster)  [unwired: 1 in, 2 out]
            n205 = Close File(refnum=w777, error in=w756) -> (error out=w750:errorcluster)  [unwired: 1 out]
            n206 = Close File(refnum=w776, error in=w755) -> (error out=w749:errorcluster)  [unwired: 1 out]
            n207 = Close File(refnum=w770, error in=w754) -> (error out=w748:errorcluster)  [unwired: 1 out]
            n208 = Close File(refnum=w769, error in=w753) -> (error out=w747:errorcluster)  [unwired: 1 out]
            n209 = Close File(refnum=w764, error in=w752) -> (error out=w746:errorcluster)  [unwired: 1 out]
            n210 = Close File(refnum=w761, error in=w751) -> (error out=w745:errorcluster)  [unwired: 1 out]
            n211 = Build Array(w750, w749, w748, w747, w746, w745) -> (w744:errorcluster[])
          }
        }
        n212 = Index Array(array=w738, index=1) -> (element=w737:string)
        n213 = String To Path(string=w737) -> (path=w662:path)
        n214 = File/Directory Info(path=w662) -> (directory=w663:bool, error out=w660:errorcluster)  [unwired: 1 in, 5 out]
        n215 = case shown="False" w663 {
          tunnel: w662 -> [w741 w742]
          tunnel: [w740 w742] -> w661
          tunnel: w660 -> [_ _]
          frame False {
            n216 = Create Folder(path (use dialog)=w741) -> (created path=w740:path)  [unwired: 1 in, 3 out]
          }
          frame True {
          }
        }
        n217 = Merge Errors(w671) -> (→"Correl files writing / closing error":errorcluster)
        n218 = Build Path(base path=w661, name or relative path="tau-U.txt" ("format string")) -> (appended path=w735:path)
        n219 = Build Path(base path=w661, name or relative path="tau-V.txt" ("format string")) -> (appended path=w725:path)
        n220 = Build Path(base path=w661, name or relative path="tau-UV.txt" ("format string")) -> (appended path=w721:path)
        n221 = Build Path(base path=w661, name or relative path="tlag.txt" ("format string")) -> (appended path=w711:path)
        n222 = Build Path(base path=w661, name or relative path="Rlag.txt" ("format string")) -> (appended path=w707:path)
        n223 = Build Path(base path=w661, name or relative path="Y.txt" ("format string")) -> (appended path=w691:path)
        n224 = call <vilib>:"Check if File or Folder Exists.vi"("path"=w735) -> ("file or folder exists?"=w734:bool, "dup path"=w732:path)  [unwired: 1 in, 8 out]
        n225 = call <vilib>:"Check if File or Folder Exists.vi"("path"=w725) -> ("file or folder exists?"=w726:bool, "dup path"=w728:path)  [unwired: 1 in, 8 out]
        n226 = call <vilib>:"Check if File or Folder Exists.vi"("path"=w721) -> ("file or folder exists?"=w720:bool, "dup path"=w718:path)  [unwired: 1 in, 8 out]
        n227 = call <vilib>:"Check if File or Folder Exists.vi"("path"=w711) -> ("file or folder exists?"=w712:bool, "dup path"=w714:path)  [unwired: 1 in, 8 out]
        n228 = call <vilib>:"Check if File or Folder Exists.vi"("path"=w707) -> ("file or folder exists?"=w706:bool, "dup path"=w704:path)  [unwired: 1 in, 8 out]
        n229 = call <vilib>:"Check if File or Folder Exists.vi"("path"=w691) -> ("file or folder exists?"=w692:bool, "dup path"=w694:path)  [unwired: 1 in, 8 out]
        n230 = case shown="False" w734 {
          tunnel: [T3."create" ("operation (0:open)") T3."replace" ("operation (0:open)")] -> w733
          tunnel: [w808 w811] -> w731
          tunnel: w732 -> [w808 w811]
          frame False {
          }
          frame True {
          }
        }
        n231 = case shown="False" w726 {
          tunnel: [T3."create" ("operation (0:open)") T3."replace" ("operation (0:open)")] -> w727
          tunnel: [w804 w806] -> w729
          tunnel: w728 -> [w804 w806]
          frame False {
          }
          frame True {
          }
        }
        n232 = case shown="False" w720 {
          tunnel: [T3."create" ("operation (0:open)") T3."replace" ("operation (0:open)")] -> w719
          tunnel: [w800 w802] -> w717
          tunnel: w718 -> [w800 w802]
          frame False {
          }
          frame True {
          }
        }
        n233 = case shown="False" w712 {
          tunnel: [T3."create" ("operation (0:open)") T3."replace" ("operation (0:open)")] -> w713
          tunnel: [w796 w798] -> w715
          tunnel: w714 -> [w796 w798]
          frame False {
          }
          frame True {
          }
        }
        n234 = case shown="False" w706 {
          tunnel: [T3."create" ("operation (0:open)") T3."replace" ("operation (0:open)")] -> w705
          tunnel: [w792 w794] -> w703
          tunnel: w704 -> [w792 w794]
          frame False {
          }
          frame True {
          }
        }
        n235 = case shown="False" w692 {
          tunnel: [T3."create" ("operation (0:open)") T3."replace" ("operation (0:open)")] -> w693
          tunnel: [w788 w790] -> w695
          tunnel: w694 -> [w788 w790]
          frame False {
          }
          frame True {
          }
        }
        n236 = Open/Create/Replace File(file path (use dialog)=w731, operation (0:open)=w733) -> (refnum out=w730:refnum<file>, error out=w677:errorcluster)  [unwired: 1 in, 4 out]
        n237 = Open/Create/Replace File(file path (use dialog)=w729, operation (0:open)=w727) -> (refnum out=w723:refnum<file>, error out=w676:errorcluster)  [unwired: 1 in, 4 out]
        n238 = Open/Create/Replace File(file path (use dialog)=w717, operation (0:open)=w719) -> (refnum out=w716:refnum<file>, error out=w675:errorcluster)  [unwired: 1 in, 4 out]
        n239 = Open/Create/Replace File(file path (use dialog)=w715, operation (0:open)=w713) -> (refnum out=w709:refnum<file>, error out=w674:errorcluster)  [unwired: 1 in, 4 out]
        n240 = Open/Create/Replace File(file path (use dialog)=w703, operation (0:open)=w705) -> (refnum out=w702:refnum<file>, error out=w673:errorcluster)  [unwired: 1 in, 4 out]
        n241 = Open/Create/Replace File(file path (use dialog)=w695, operation (0:open)=w693) -> (refnum out=w689:refnum<file>, error out=w672:errorcluster)  [unwired: 1 in, 4 out]
        n242 = Build Array(w677, w676, w675, w674, w673, w672) -> (w665:errorcluster[])
        n243 = Merge Errors(w665) -> (→"Correl files creation error":errorcluster)
      }
    }
    n244 = Increment(x=w540) -> (x+1=→"Current row no.":i32)
    n245 = Merge Errors(w544, w543, w542) -> (→"stats file error":errorcluster)
  }
  n246 = Array Size(array=w116) -> (size(s)=w92:i32[])
  n247 = Index Array(array=w92, index=0) -> (element=→"No. of rows":i32)
  n248 = Transpose 2D Array(2D array=w33) -> (transposed array=w34:dbl[][])
  n249 = Transpose 2D Array(2D array=w32) -> (transposed array=w39:dbl[][])
  n250 = Transpose 2D Array(2D array=w31) -> (transposed array=w41:dbl[][])
  n251 = Transpose 2D Array(2D array=w30) -> (transposed array=w45:dbl[][])
  n252 = Transpose 2D Array(2D array=w21) -> (transposed array=w48:dbl[][])
  n253 = Transpose 2D Array(2D array=w29) -> (transposed array=w51:dbl[][])
  n254 = Array To Spreadsheet String(array=w34, 3:w22) -> (spreadsheet string=w35:string)  [unwired: 1 out]
  n255 = Array To Spreadsheet String(array=w39, 3:w22) -> (spreadsheet string=w36:string)  [unwired: 1 out]
  n256 = Array To Spreadsheet String(array=w41, 3:w22) -> (spreadsheet string=w40:string)  [unwired: 1 out]
  n257 = Array To Spreadsheet String(array=w45, 3:w22) -> (spreadsheet string=w44:string)  [unwired: 1 out]
  n258 = Array To Spreadsheet String(array=w48, 3:w22) -> (spreadsheet string=w46:string)  [unwired: 1 out]
  n259 = Array To Spreadsheet String(array=w51, 3:w22) -> (spreadsheet string=w50:string)  [unwired: 1 out]
  n260 = Write to Text File(file (use dialog)=w28, text=w35) -> (refnum out=w37:refnum<file>)  [unwired: 1 in, 3 out]
  n261 = Write to Text File(file (use dialog)=w27, text=w36) -> (refnum out=w38:refnum<file>)  [unwired: 1 in, 3 out]
  n262 = Write to Text File(file (use dialog)=w26, text=w40) -> (refnum out=w42:refnum<file>)  [unwired: 1 in, 3 out]
  n263 = Write to Text File(file (use dialog)=w25, text=w44) -> (refnum out=w43:refnum<file>)  [unwired: 1 in, 3 out]
  n264 = Write to Text File(file (use dialog)=w24, text=w46) -> (refnum out=w47:refnum<file>)  [unwired: 1 in, 3 out]
  n265 = Write to Text File(file (use dialog)=w23, text=w50) -> (refnum out=w49:refnum<file>)  [unwired: 1 in, 3 out]
  n266 = Close File(refnum=w37) -> ()  [unwired: 1 in, 2 out]
  n267 = Close File(refnum=w38) -> ()  [unwired: 1 in, 2 out]
  n268 = Close File(refnum=w42) -> ()  [unwired: 1 in, 2 out]
  n269 = Close File(refnum=w43) -> ()  [unwired: 1 in, 2 out]
  n270 = Close File(refnum=w47) -> ()  [unwired: 1 in, 2 out]
  n271 = Close File(refnum=w49) -> ()  [unwired: 1 in, 2 out]
  n272 = Close File(refnum=w20, error in=w19) -> (error out=w55:errorcluster)  [unwired: 1 out]
  n273 = Close File(refnum=w18, error in=w17) -> (error out=w54:errorcluster)  [unwired: 1 out]
  n274 = Close File(refnum=w16, error in=w15) -> (error out=w53:errorcluster)  [unwired: 1 out]
  n275 = Merge Errors(w55, w54, w53) -> (→"Final error":errorcluster)
